vi "Write Flow Control Settings.vi"(10 "Flow Control Settings":T1={"DAC Channel"=1, "ROT Bias"=65} {"ROT Bias" max=127 step=1; "DAC Channel" min=1 max=4 step=1}, 11 "FlowControlActuator in":refnum<class "FlowControlActuator.lvclass">) -> (3 "FlowControlActuator out":refnum<class "FlowControlActuator.lvclass">)   [LabVIEW 2015, in "FlowControlActuator.lvclass"]
uses:
  FlowControlActuator.lvclass
  Typedefs/Flow Control Settings.ctl
  FlowControlActuator.lvclass/FlowControlActuator.ctl
  Typedefs/FAMTTypedefs.lvlib
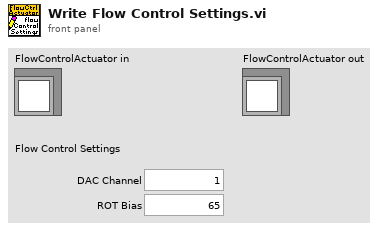
[diagram p1: front panel]
types:
  T1 = typedef "FAMTTypedefs.lvlib/Flow Control Settings.ctl" = cluster{"DAC Channel":u8, "ROT Bias":u8}
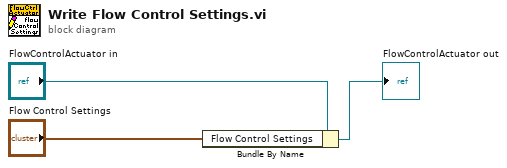
[diagram p0: block diagram]
diagram:
  n1 = Bundle By Name(cluster="FlowControlActuator in", "Flow Control Settings"="Flow Control Settings") -> (→"FlowControlActuator out":refnum<class "FlowControlActuator.lvclass">)
